vi "Data Plopper.vi"(11 "Roughness":T1) -> ()   [LabVIEW 2018]
panel:
  out "Peak density":dbl(graph)
  out "Slopes":cluster{"Rdq":dbl, "Rda":dbl}(graph)
  out "RzDIN/RzJIS":cluster{"RzDIN":dbl, "RzJIS":dbl}(graph)
  out "Kurtosis":dbl(graph)
  out "Skewdness":dbl(graph)
  out "Global Heuristics":T2(graph)
  out "Averages":T3(graph)
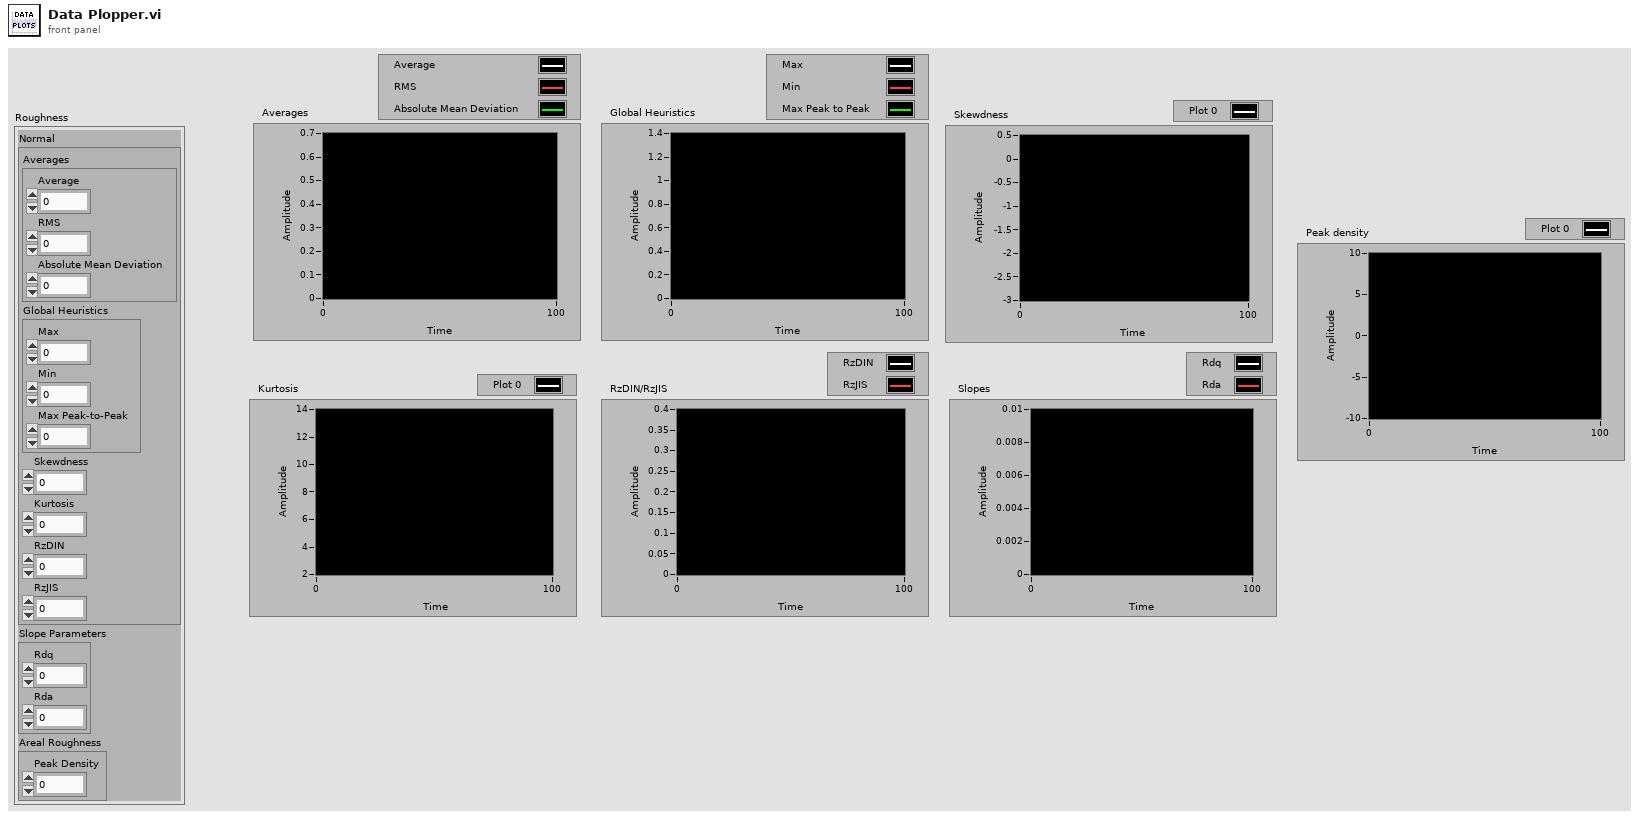
[diagram p1: front panel]
types:
  T1 = cluster{"Normal":cluster{"Averages":cluster{"Average":dbl, "RMS":dbl, "Absolute Mean Deviation":dbl}, "Global Heuristics":cluster{"Max":dbl, "Min":dbl, "Max Peak-to-Peak":dbl}, "Skewdness":dbl, "Kurtosis":dbl, "RzDIN":dbl, "RzJIS":dbl}, "Slope Parameters":cluster{"Rdq":dbl, "Rda":dbl}, "Areal Roughness":cluster{"Peak Density":dbl}}
  T2 = cluster{"Max":dbl, "Min":dbl, "Max Peak-to-Peak":dbl}
  T3 = cluster{"Average":dbl, "RMS":dbl, "Absolute Mean Deviation":dbl}
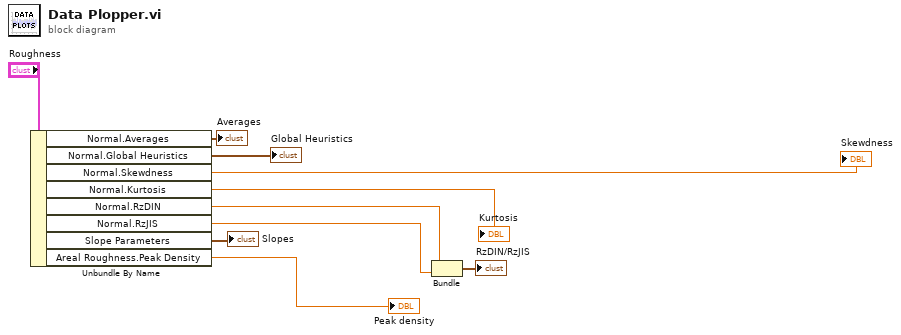
[diagram p0: block diagram]
diagram:
  n1 = Unbundle By Name("Roughness") -> ("Normal.Averages"=→"Averages":T3, "Normal.Global Heuristics"=→"Global Heuristics":T2, "Normal.Skewdness"=→"Skewdness":dbl, "Normal.Kurtosis"=→"Kurtosis":dbl, "Normal.RzDIN"=w4:dbl, "Normal.RzJIS"=w3:dbl, "Slope Parameters"=→"Slopes":cluster{"Rdq":dbl, "Rda":dbl}, "Areal Roughness.Peak Density"=→"Peak density":dbl)
  n2 = Bundle("RzDIN"=w4, "RzJIS"=w3) -> (→"RzDIN/RzJIS":cluster{"RzDIN":dbl, "RzJIS":dbl})  [unwired: 1 in]
